vi "rs3 Set Advanced Depth.vi"(0 "Depth Presets":T1(ring), 1 "device in":u64=370866768, 3 "error in (no error)":errorcluster) -> (4 "Set advanced error":string, 5 "Dev out":u64=370866768, 6 "error out":errorcluster)   [LabVIEW 2017, in "libRealSense3.lvlib"]
doc: "The RealSense D4xx cameras are based on a stereo algorithm that has been accelerated as a fixed-function inside an ASIC. There are many parameters that affect the calculation of the depth. The basic task is to solve the correspondance problem - i.e. figure out which patches in the left image match up to those in the right image by doing a search along an epipolar line (x-axis). The x-axis difference for each object point is known as the disparity. \n\nIn general depth can be estimated for most points in the scene, but some points will have a very low confidence because 1. they are may be occluded (not seen by both imagers), or 2. have very little texture on them which will lead to an ambiquity (ex. when looking at a completely uniform white wall it, there are no best correspondances).\n\nThis VI allows you to set the many parameters that affect the algorith, as well as the color reproduction. \nNote that the color correction matrix will NOT have any effect on the depth calculations."
uses:
  libRealSense3.lvlib
panel:
  # "RS3 Set Advanced Depth"
  # "(C) 2020 Intel Corp.,  AGJ"
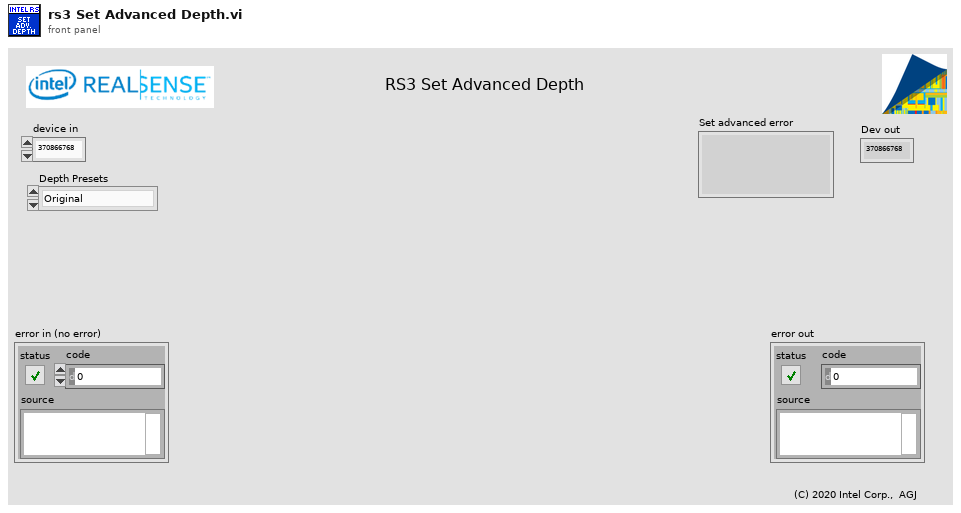
[diagram p1: front panel]
types:
  T1 = enum16{"Original", "High Density", "Medium Density", "High Accuracy", "Hand", "Short Range", "Flat wall"}
  T2 = cluster{"lambdaCensus":sgl, "lambdaAD":sgl, "ignoreSAD":u32}
  T3 = cluster{"depth control":cluster{"plusIncrement":u32, "MinusDecrement":u32, "deepSeaMedianThreshold":u32, "scoreThreshA":u32, "scoreThreshB":u32, "textureDifferenceThreshold":u32, "textureCountThreshold":u32, "deepSeaSecondPeakThreshold":u32, "deepSeaNeighborThreshold":u32, "IrAgreeThreshold":u32}, "STColorCorrection output":cluster{"colorCorrection 1":sgl, "colorCorrection 2":sgl, "colorCorrection 3":sgl, "colorCorrection 4":sgl, "colorCorrection 5":sgl, "colorCorrection 6":sgl, "colorCorrection 7":sgl, "colorCorrection 8":sgl, "colorCorrection 9":sgl, "colorCorrection 10":sgl, "colorCorrection 11":sgl, "colorCorrection 12":sgl}, "HDAD":cluster{"lambdaCensus":sgl, "lambdaAD":sgl, "ignoreSAD":u32}, "ST RSM":cluster{"rsmBypass":u32, "diffThresh":sgl, "sloRauDiffThresh":sgl, "removeThresh":u32}, "ST SLO Penalty":cluster{"sloK1Penalty":u32, "sloK2Penalty":u32, "sloK1PenaltyMod1":u32, "sloK2PenaltyMod1":u32, "sloK1PenaltyMod2":u32, "sloK2PenaltyMod2":u32}, "ST SLO Threshold":cluster{"SLOdiffThresholdRed":u32, "SLODiffThresholdGreen":u32, "SLODiffThresholdBlue":u32}, "ST Rau Threshold":cluster{"rauDiffThresholdRed":u32, "rauDiffThresholdGreen":u32, "rauDiffThresholdBlue":u32}, "ST Color Control":cluster{"disableSADColor":u32, "disableRAUColor":u32, "disableSLORightColor":u32, "disableSLOLeftColor":u32, "disableSADNormalize":u32}, "ST RAU vector":cluster{"minWest":u32, "minEast":u32, "minWEsum":u32, "minNorth":u32, "minSouth":u32, "minNSSum":u32, "uStrink":u32, "vShrink":u32}, "Depth Table":cluster{"depthUnits, um":u32, "depthClampMin":u32, "depthClampMax":u32, "disparityMultiplier":u32, "disparityShift":u32}, "ST_AE_Control":cluster{"meanIntensitySetpoint":u32}, "ST_CensusEnable":cluster{"uDiameter":u32, "vDiameter":u32}}
  T4 = cluster{"depthUnits, um":u32, "depthClampMin":u32, "depthClampMax":u32, "disparityMultiplier":u32, "disparityShift(0-127)":u32}
  T5 = cluster{"minWest (60)":u32, "minEast (61)":u32, "minWEsum (62)":u32, "minNorth (63)":u32, "minSouth (64)":u32, "minNSSum(65)":u32, "uStrink (66)":u32, "vShrink (67)":u32}
  T6 = cluster{"rauDiffThreshRed(73)":u32, "rauDiffThreshGreen(74)":u32, "rauDiffThreshBlue(75)":u32}
  T7 = cluster{"sloK1Penalty (79)":u32, "sloK2Penalty (80)":u32, "sloK1PenaltyMod1(81)":u32, "sloK2PenaltyMod1(82)":u32, "sloK1PenaltyMod2(83)":u32, "sloK2PenaltyMod2(84)":u32}
  T8 = cluster{"SLOdiffThreshRed(76)":u32, "SLODiffThreshGreen(77)":u32, "SLODiffThreshBlue(78)":u32}
  T9 = cluster{"disableSADColor(68)":u32, "disableRAUColor(69)":u32, "disableSLORightColor(70)":u32, "disableSLOLeftColor(71)":u32, "disableSADNormalize(72)":u32}
  T10 = cluster{"rsmBypass (56)":u32, "diffThresh (57)":sgl, "sloRauDiffThresh(58)":sgl, "removeThresh(59)":u32}
  T11 = cluster{"plusIncrement (47)":u32, "MinusDecrement (46)":u32, "deepSeaMedianThreshold (48)":u32, "scoreThreshA(49)":u32, "scoreThreshB (50)":u32, "textureDifferenceThreshold (52)":u32, "textureCountThreshold (51)":u32, "deepSea2ndPeakThresh.(53)":u32, "deepSeaNeighborThresh.(54)":u32, "LRAgreeThreshold (55)":u32}
  T12 = cluster{"plusIncrement":u32, "MinusDecrement":u32, "deepSeaMedianThreshold":u32, "scoreThreshA":u32, "scoreThreshB":u32, "textureDifferenceThreshold":u32, "textureCountThreshold":u32, "deepSeaSecondPeakThreshold":u32, "deepSeaNeighborThreshold":u32, "IrAgreeThreshold":u32}
  T13 = cluster{"rsmBypass":u32, "diffThresh":sgl, "sloRauDiffThresh":sgl, "removeThresh":u32}
  T14 = cluster{"sloK1Penalty":u32, "sloK2Penalty":u32, "sloK1PenaltyMod1":u32, "sloK2PenaltyMod1":u32, "sloK1PenaltyMod2":u32, "sloK2PenaltyMod2":u32}
  T15 = cluster{"SLOdiffThresholdRed":u32, "SLODiffThresholdGreen":u32, "SLODiffThresholdBlue":u32}
  T16 = cluster{"rauDiffThresholdRed":u32, "rauDiffThresholdGreen":u32, "rauDiffThresholdBlue":u32}
  T17 = cluster{"disableSADColor":u32, "disableRAUColor":u32, "disableSLORightColor":u32, "disableSLOLeftColor":u32, "disableSADNormalize":u32}
  T18 = cluster{"minWest":u32, "minEast":u32, "minWEsum":u32, "minNorth":u32, "minSouth":u32, "minNSSum":u32, "uStrink":u32, "vShrink":u32}
  T19 = cluster{"depthUnits, um":u32, "depthClampMin":u32, "depthClampMax":u32, "disparityMultiplier":u32, "disparityShift":u32}
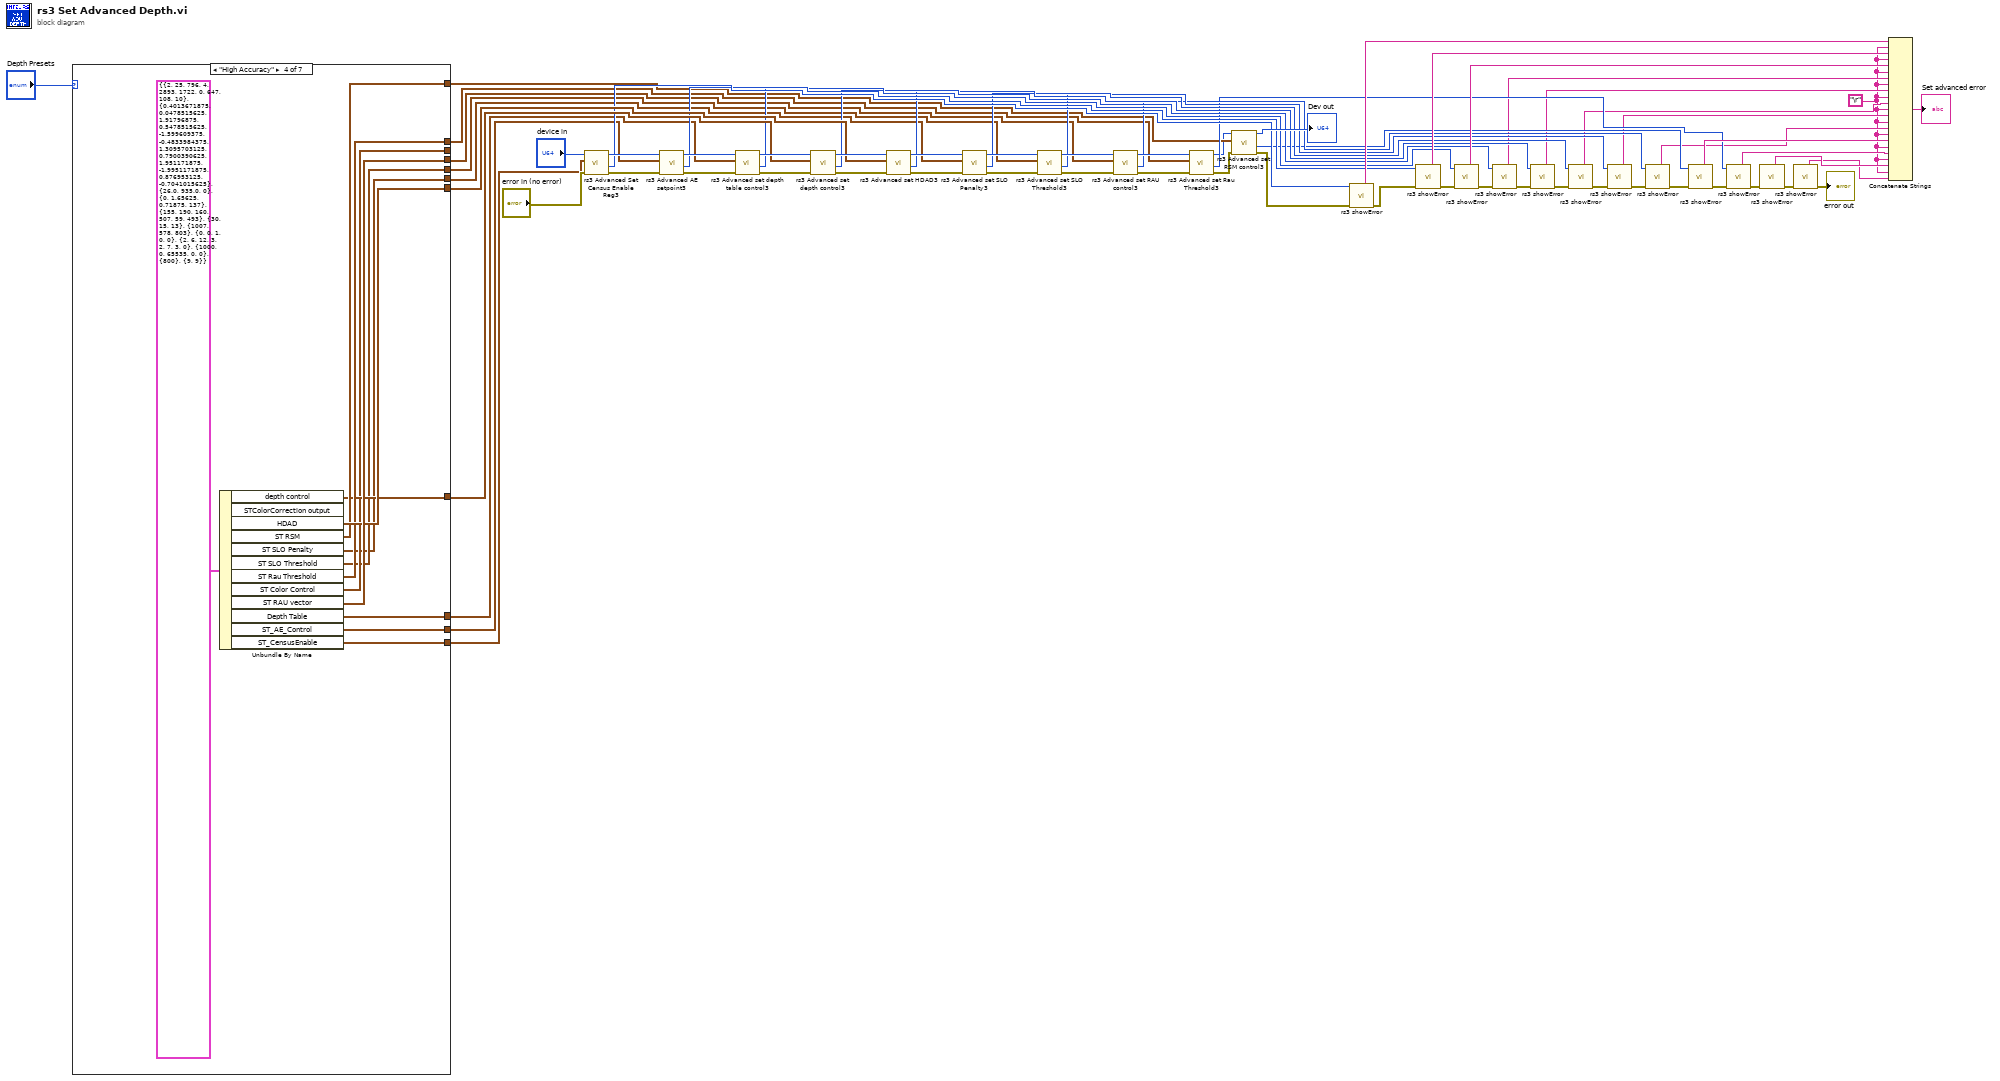
[diagram p0: block diagram]
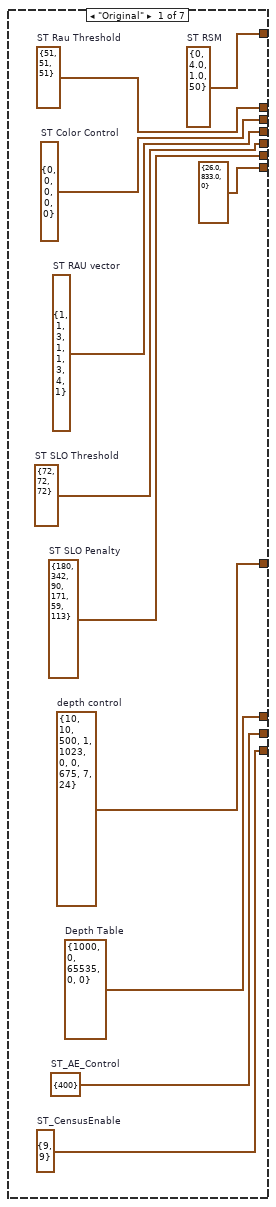
[diagram p2: hidden frame]
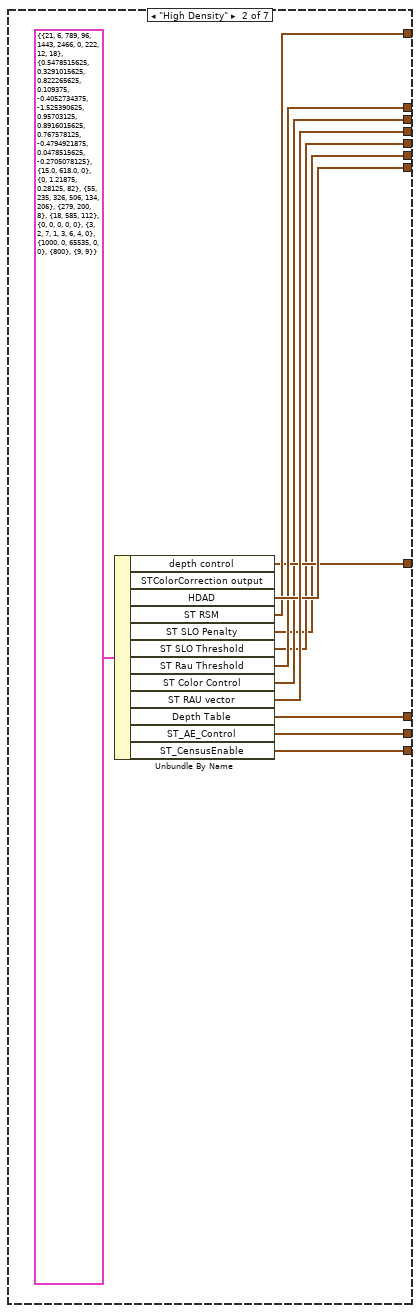
[diagram p3: hidden frame]
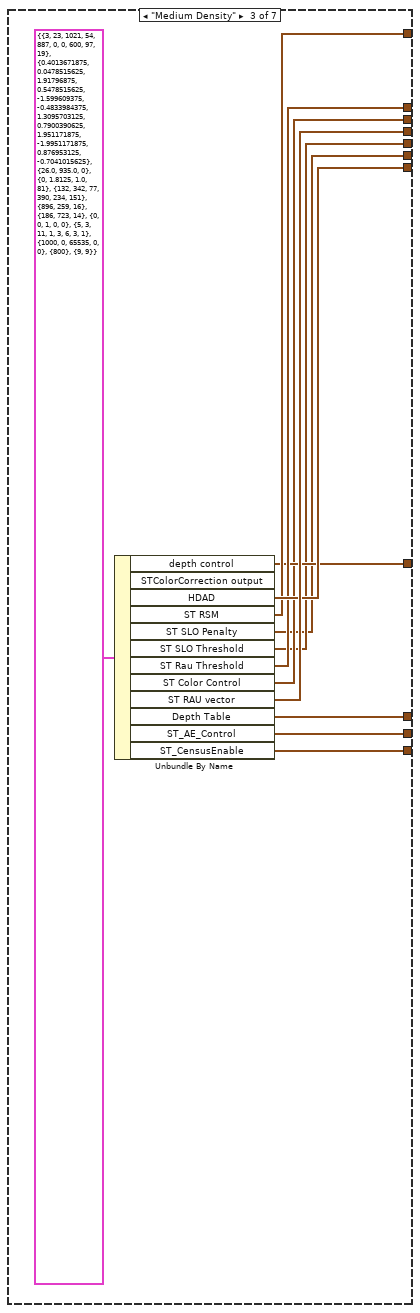
[diagram p4: hidden frame]
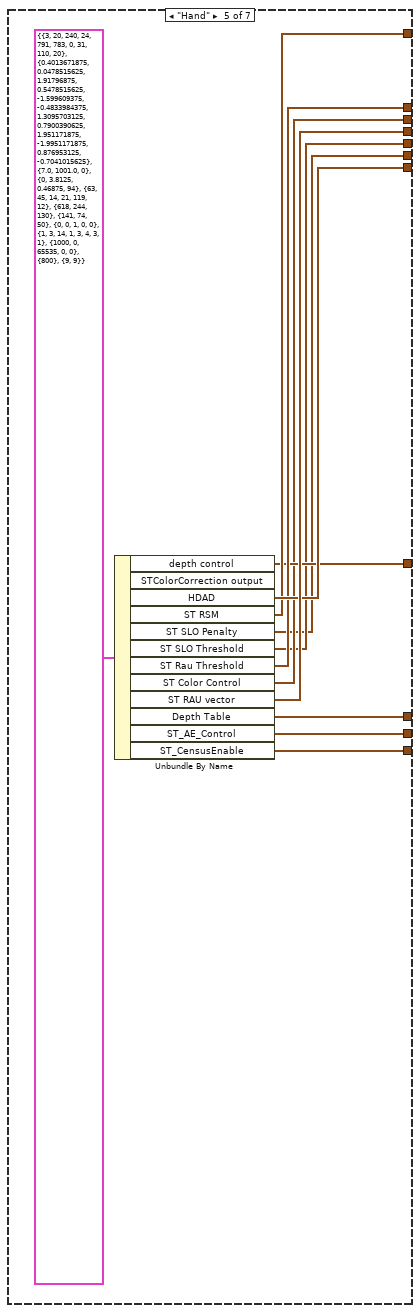
[diagram p5: hidden frame]
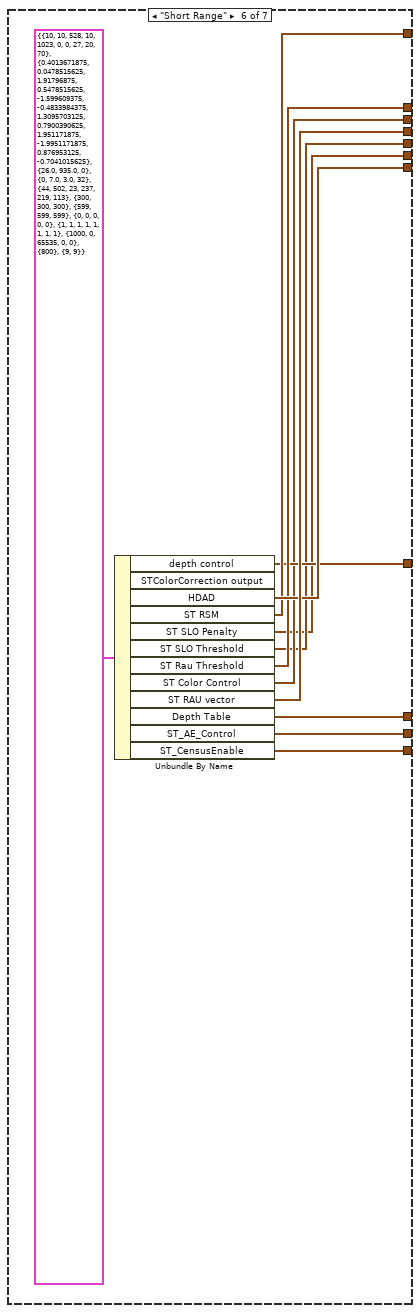
[diagram p6: hidden frame]
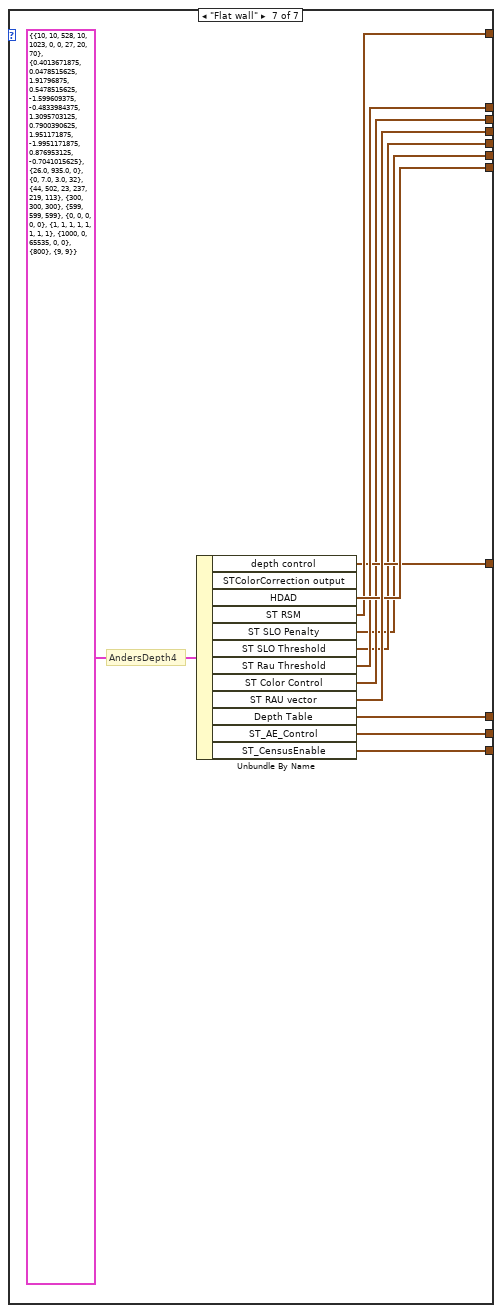
[diagram p7: hidden frame]
diagram:
  w25 = "\r"
  n1 = case shown="\"High Accuracy\"" "Depth Presets" {
    tunnel: [w79 w84 w97 w109 w121 w133 w145] -> w49
    tunnel: [w78 w89 w102 w114 w126 w138 w150] -> w19
    tunnel: [w73 w91 w104 w116 w128 w140 w152] -> w20
    tunnel: [w74 w87 w100 w112 w124 w136 w148] -> w21
    tunnel: [w77 w83 w96 w108 w120 w132 w144] -> _
    tunnel: [w76 w82 w95 w107 w119 w131 w143] -> w22
    tunnel: [w75 w81 w94 w106 w118 w130 w142] -> w23
    tunnel: [T2 {"lambdaCensus"=26.0, "lambdaAD"=833.0, "ignoreSAD"=0} ("HDAD 2") w90 w103 w115 w127 w139 w151] -> w48
    tunnel: [w70 w85 w98 w110 w122 w134 w146] -> w17
    tunnel: [w71 w86 w99 w111 w123 w135 w147] -> w18
    tunnel: [w72 w88 w101 w113 w125 w137 w149] -> w16
    frame "Original" {
      w71 = cluster{"uDiameter":u32, "vDiameter":u32} {"uDiameter"=9, "vDiameter"=9}  # ST_CensusEnable
      w72 = T4 {"depthUnits, um"=1000, "depthClampMin"=0, "depthClampMax"=65535, "disparityMultiplier"=0, "disparityShift(0-127)"=0}  # Depth Table
      w70 = cluster{"meanIntensitySetpoint":u32} {"meanIntensitySetpoint"=400}  # ST_AE_Control
      w73 = T5 {"minWest (60)"=1, "minEast (61)"=1, "minWEsum (62)"=3, "minNorth (63)"=1, "minSouth (64)"=1, "minNSSum(65)"=3, "uStrink (66)"=4, "vShrink (67)"=1}  # ST RAU vector
      w74 = T6 {"rauDiffThreshRed(73)"=51, "rauDiffThreshGreen(74)"=51, "rauDiffThreshBlue(75)"=51}  # ST Rau Threshold
      w75 = T7 {"sloK1Penalty (79)"=180, "sloK2Penalty (80)"=342, "sloK1PenaltyMod1(81)"=90, "sloK2PenaltyMod1(82)"=171, "sloK1PenaltyMod2(83)"=59, "sloK2PenaltyMod2(84)"=113}  # ST SLO Penalty
      w76 = T8 {"SLOdiffThreshRed(76)"=72, "SLODiffThreshGreen(77)"=72, "SLODiffThreshBlue(78)"=72}  # ST SLO Threshold
      w77 = T9 {"disableSADColor(68)"=0, "disableRAUColor(69)"=0, "disableSLORightColor(70)"=0, "disableSLOLeftColor(71)"=0, "disableSADNormalize(72)"=0}  # ST Color Control
      w78 = T10 {"rsmBypass (56)"=0, "diffThresh (57)"=4.0, "sloRauDiffThresh(58)"=1.0, "removeThresh(59)"=50}  # ST RSM
      w79 = T11 {"plusIncrement (47)"=10, "MinusDecrement (46)"=10, "deepSeaMedianThreshold (48)"=500, "scoreThreshA(49)"=1, "scoreThreshB (50)"=1023, "textureDifferenceThreshold (52)"=0, "textureCountThreshold (51)"=0, "deepSea2ndPeakThresh.(53)"=675, "deepSeaNeighborThresh.(54)"=7, "LRAgreeThreshold (55)"=24}  # depth control
    }
    frame "High Density" {
      n2 = Unbundle By Name(T3 {"depth control"={"plusIncrement"=21, "MinusDecrement"=6, "deepSeaMedianThreshold"=789, "scoreThreshA"=96, "scoreThreshB"=1443, "textureDifferenceThreshold"=2466, "textureCountThreshold"=0, "deepSeaSecondPeakThreshold"=222, "deepSeaNeighborThreshold"=12, "IrAgreeThreshold"=18}, "STColorCorrection output"={"colorCorrection 1"=0.54785156, "colorCorrection 2"=0.32910156, "colorCorrection 3"=0.8222656, "colorCorrection 4"=0.109375, "colorCorrection 5"=-0.40527344, "colorCorrection 6"=-1.5253906, "colorCorrection 7"=0.95703125, "colorCorrection 8"=0.89160156, "colorCorrection 9"=0.7675781, "colorCorrection 10"=-0.4794922, "colorCorrection 11"=0.047851562, "colorCorrection 12"=-0.2705078}, "HDAD"={"lambdaCensus"=15.0, "lambdaAD"=618.0, "ignoreSAD"=0}, "ST RSM"={"rsmBypass"=0, "diffThresh"=1.21875, "sloRauDiffThresh"=0.28125, "removeThresh"=82}, "ST SLO Penalty"={"sloK1Penalty"=55, "sloK2Penalty"=235, "sloK1PenaltyMod1"=326, "sloK2PenaltyMod1"=506, "sloK1PenaltyMod2"=134, "sloK2PenaltyMod2"=206}, "ST SLO Threshold"={"SLOdiffThresholdRed"=279, "SLODiffThresholdGreen"=200, "SLODiffThresholdBlue"=8}, "ST Rau Threshold"={"rauDiffThresholdRed"=18, "rauDiffThresholdGreen"=585, "rauDiffThresholdBlue"=112}, "ST Color Control"={"disableSADColor"=0, "disableRAUColor"=0, "disableSLORightColor"=0, "disableSLOLeftColor"=0, "disableSADNormalize"=0}, "ST RAU vector"={"minWest"=3, "minEast"=2, "minWEsum"=7, "minNorth"=1, "minSouth"=3, "minNSSum"=6, "uStrink"=4, "vShrink"=0}, "Depth Table"={"depthUnits, um"=1000, "depthClampMin"=0, "depthClampMax"=65535, "disparityMultiplier"=0, "disparityShift"=0}, "ST_AE_Control"={"meanIntensitySetpoint"=800}, "ST_CensusEnable"={"uDiameter"=9, "vDiameter"=9}} ("depth settings 2")) -> ("depth control"=w84:T12, "HDAD"=w90:T2, "ST RSM"=w89:T13, "ST SLO Penalty"=w81:T14, "ST SLO Threshold"=w82:T15, "ST Rau Threshold"=w87:T16, "ST Color Control"=w83:T17, "ST RAU vector"=w91:T18, "Depth Table"=w88:T19, "ST_AE_Control"=w85:cluster{"meanIntensitySetpoint":u32}, "ST_CensusEnable"=w86:cluster{"uDiameter":u32, "vDiameter":u32})  [unwired: 1 out]
    }
    frame "Medium Density" {
      n3 = Unbundle By Name(T3 {"depth control"={"plusIncrement"=3, "MinusDecrement"=23, "deepSeaMedianThreshold"=1021, "scoreThreshA"=54, "scoreThreshB"=887, "textureDifferenceThreshold"=0, "textureCountThreshold"=0, "deepSeaSecondPeakThreshold"=600, "deepSeaNeighborThreshold"=97, "IrAgreeThreshold"=19}, "STColorCorrection output"={"colorCorrection 1"=0.4013672, "colorCorrection 2"=0.047851562, "colorCorrection 3"=1.9179688, "colorCorrection 4"=0.54785156, "colorCorrection 5"=-1.5996094, "colorCorrection 6"=-0.48339844, "colorCorrection 7"=1.3095703, "colorCorrection 8"=0.79003906, "colorCorrection 9"=1.9511719, "colorCorrection 10"=-1.9951172, "colorCorrection 11"=0.8769531, "colorCorrection 12"=-0.70410156}, "HDAD"={"lambdaCensus"=26.0, "lambdaAD"=935.0, "ignoreSAD"=0}, "ST RSM"={"rsmBypass"=0, "diffThresh"=1.8125, "sloRauDiffThresh"=1.0, "removeThresh"=81}, "ST SLO Penalty"={"sloK1Penalty"=132, "sloK2Penalty"=342, "sloK1PenaltyMod1"=77, "sloK2PenaltyMod1"=390, "sloK1PenaltyMod2"=234, "sloK2PenaltyMod2"=151}, "ST SLO Threshold"={"SLOdiffThresholdRed"=896, "SLODiffThresholdGreen"=259, "SLODiffThresholdBlue"=16}, "ST Rau Threshold"={"rauDiffThresholdRed"=186, "rauDiffThresholdGreen"=723, "rauDiffThresholdBlue"=14}, "ST Color Control"={"disableSADColor"=0, "disableRAUColor"=0, "disableSLORightColor"=1, "disableSLOLeftColor"=0, "disableSADNormalize"=0}, "ST RAU vector"={"minWest"=5, "minEast"=3, "minWEsum"=11, "minNorth"=1, "minSouth"=3, "minNSSum"=6, "uStrink"=3, "vShrink"=1}, "Depth Table"={"depthUnits, um"=1000, "depthClampMin"=0, "depthClampMax"=65535, "disparityMultiplier"=0, "disparityShift"=0}, "ST_AE_Control"={"meanIntensitySetpoint"=800}, "ST_CensusEnable"={"uDiameter"=9, "vDiameter"=9}} ("depth settings 2")) -> ("depth control"=w97:T12, "HDAD"=w103:T2, "ST RSM"=w102:T13, "ST SLO Penalty"=w94:T14, "ST SLO Threshold"=w95:T15, "ST Rau Threshold"=w100:T16, "ST Color Control"=w96:T17, "ST RAU vector"=w104:T18, "Depth Table"=w101:T19, "ST_AE_Control"=w98:cluster{"meanIntensitySetpoint":u32}, "ST_CensusEnable"=w99:cluster{"uDiameter":u32, "vDiameter":u32})  [unwired: 1 out]
    }
    frame "High Accuracy" {
      n4 = Unbundle By Name(T3 {"depth control"={"plusIncrement"=2, "MinusDecrement"=25, "deepSeaMedianThreshold"=796, "scoreThreshA"=4, "scoreThreshB"=2893, "textureDifferenceThreshold"=1722, "textureCountThreshold"=0, "deepSeaSecondPeakThreshold"=647, "deepSeaNeighborThreshold"=108, "IrAgreeThreshold"=10}, "STColorCorrection output"={"colorCorrection 1"=0.4013672, "colorCorrection 2"=0.047851562, "colorCorrection 3"=1.9179688, "colorCorrection 4"=0.54785156, "colorCorrection 5"=-1.5996094, "colorCorrection 6"=-0.48339844, "colorCorrection 7"=1.3095703, "colorCorrection 8"=0.79003906, "colorCorrection 9"=1.9511719, "colorCorrection 10"=-1.9951172, "colorCorrection 11"=0.8769531, "colorCorrection 12"=-0.70410156}, "HDAD"={"lambdaCensus"=26.0, "lambdaAD"=935.0, "ignoreSAD"=0}, "ST RSM"={"rsmBypass"=0, "diffThresh"=1.65625, "sloRauDiffThresh"=0.71875, "removeThresh"=137}, "ST SLO Penalty"={"sloK1Penalty"=155, "sloK2Penalty"=190, "sloK1PenaltyMod1"=160, "sloK2PenaltyMod1"=507, "sloK1PenaltyMod2"=59, "sloK2PenaltyMod2"=493}, "ST SLO Threshold"={"SLOdiffThresholdRed"=30, "SLODiffThresholdGreen"=15, "SLODiffThresholdBlue"=13}, "ST Rau Threshold"={"rauDiffThresholdRed"=1007, "rauDiffThresholdGreen"=578, "rauDiffThresholdBlue"=803}, "ST Color Control"={"disableSADColor"=0, "disableRAUColor"=0, "disableSLORightColor"=1, "disableSLOLeftColor"=0, "disableSADNormalize"=0}, "ST RAU vector"={"minWest"=2, "minEast"=6, "minWEsum"=12, "minNorth"=3, "minSouth"=2, "minNSSum"=7, "uStrink"=3, "vShrink"=0}, "Depth Table"={"depthUnits, um"=1000, "depthClampMin"=0, "depthClampMax"=65535, "disparityMultiplier"=0, "disparityShift"=0}, "ST_AE_Control"={"meanIntensitySetpoint"=800}, "ST_CensusEnable"={"uDiameter"=9, "vDiameter"=9}} ("depth settings 2")) -> ("depth control"=w109:T12, "HDAD"=w115:T2, "ST RSM"=w114:T13, "ST SLO Penalty"=w106:T14, "ST SLO Threshold"=w107:T15, "ST Rau Threshold"=w112:T16, "ST Color Control"=w108:T17, "ST RAU vector"=w116:T18, "Depth Table"=w113:T19, "ST_AE_Control"=w110:cluster{"meanIntensitySetpoint":u32}, "ST_CensusEnable"=w111:cluster{"uDiameter":u32, "vDiameter":u32})  [unwired: 1 out]
    }
    frame "Hand" {
      n5 = Unbundle By Name(T3 {"depth control"={"plusIncrement"=3, "MinusDecrement"=20, "deepSeaMedianThreshold"=240, "scoreThreshA"=24, "scoreThreshB"=791, "textureDifferenceThreshold"=783, "textureCountThreshold"=0, "deepSeaSecondPeakThreshold"=31, "deepSeaNeighborThreshold"=110, "IrAgreeThreshold"=20}, "STColorCorrection output"={"colorCorrection 1"=0.4013672, "colorCorrection 2"=0.047851562, "colorCorrection 3"=1.9179688, "colorCorrection 4"=0.54785156, "colorCorrection 5"=-1.5996094, "colorCorrection 6"=-0.48339844, "colorCorrection 7"=1.3095703, "colorCorrection 8"=0.79003906, "colorCorrection 9"=1.9511719, "colorCorrection 10"=-1.9951172, "colorCorrection 11"=0.8769531, "colorCorrection 12"=-0.70410156}, "HDAD"={"lambdaCensus"=7.0, "lambdaAD"=1001.0, "ignoreSAD"=0}, "ST RSM"={"rsmBypass"=0, "diffThresh"=3.8125, "sloRauDiffThresh"=0.46875, "removeThresh"=94}, "ST SLO Penalty"={"sloK1Penalty"=63, "sloK2Penalty"=45, "sloK1PenaltyMod1"=14, "sloK2PenaltyMod1"=21, "sloK1PenaltyMod2"=119, "sloK2PenaltyMod2"=12}, "ST SLO Threshold"={"SLOdiffThresholdRed"=618, "SLODiffThresholdGreen"=244, "SLODiffThresholdBlue"=130}, "ST Rau Threshold"={"rauDiffThresholdRed"=141, "rauDiffThresholdGreen"=74, "rauDiffThresholdBlue"=50}, "ST Color Control"={"disableSADColor"=0, "disableRAUColor"=0, "disableSLORightColor"=1, "disableSLOLeftColor"=0, "disableSADNormalize"=0}, "ST RAU vector"={"minWest"=1, "minEast"=3, "minWEsum"=14, "minNorth"=1, "minSouth"=3, "minNSSum"=4, "uStrink"=3, "vShrink"=1}, "Depth Table"={"depthUnits, um"=1000, "depthClampMin"=0, "depthClampMax"=65535, "disparityMultiplier"=0, "disparityShift"=0}, "ST_AE_Control"={"meanIntensitySetpoint"=800}, "ST_CensusEnable"={"uDiameter"=9, "vDiameter"=9}} ("depth settings 2")) -> ("depth control"=w121:T12, "HDAD"=w127:T2, "ST RSM"=w126:T13, "ST SLO Penalty"=w118:T14, "ST SLO Threshold"=w119:T15, "ST Rau Threshold"=w124:T16, "ST Color Control"=w120:T17, "ST RAU vector"=w128:T18, "Depth Table"=w125:T19, "ST_AE_Control"=w122:cluster{"meanIntensitySetpoint":u32}, "ST_CensusEnable"=w123:cluster{"uDiameter":u32, "vDiameter":u32})  [unwired: 1 out]
    }
    frame "Short Range" {
      n6 = Unbundle By Name(T3 {"depth control"={"plusIncrement"=10, "MinusDecrement"=10, "deepSeaMedianThreshold"=528, "scoreThreshA"=10, "scoreThreshB"=1023, "textureDifferenceThreshold"=0, "textureCountThreshold"=0, "deepSeaSecondPeakThreshold"=27, "deepSeaNeighborThreshold"=20, "IrAgreeThreshold"=70}, "STColorCorrection output"={"colorCorrection 1"=0.4013672, "colorCorrection 2"=0.047851562, "colorCorrection 3"=1.9179688, "colorCorrection 4"=0.54785156, "colorCorrection 5"=-1.5996094, "colorCorrection 6"=-0.48339844, "colorCorrection 7"=1.3095703, "colorCorrection 8"=0.79003906, "colorCorrection 9"=1.9511719, "colorCorrection 10"=-1.9951172, "colorCorrection 11"=0.8769531, "colorCorrection 12"=-0.70410156}, "HDAD"={"lambdaCensus"=26.0, "lambdaAD"=935.0, "ignoreSAD"=0}, "ST RSM"={"rsmBypass"=0, "diffThresh"=7.0, "sloRauDiffThresh"=3.0, "removeThresh"=32}, "ST SLO Penalty"={"sloK1Penalty"=44, "sloK2Penalty"=502, "sloK1PenaltyMod1"=23, "sloK2PenaltyMod1"=237, "sloK1PenaltyMod2"=219, "sloK2PenaltyMod2"=113}, "ST SLO Threshold"={"SLOdiffThresholdRed"=300, "SLODiffThresholdGreen"=300, "SLODiffThresholdBlue"=300}, "ST Rau Threshold"={"rauDiffThresholdRed"=599, "rauDiffThresholdGreen"=599, "rauDiffThresholdBlue"=599}, "ST Color Control"={"disableSADColor"=0, "disableRAUColor"=0, "disableSLORightColor"=0, "disableSLOLeftColor"=0, "disableSADNormalize"=0}, "ST RAU vector"={"minWest"=1, "minEast"=1, "minWEsum"=1, "minNorth"=1, "minSouth"=1, "minNSSum"=1, "uStrink"=1, "vShrink"=1}, "Depth Table"={"depthUnits, um"=1000, "depthClampMin"=0, "depthClampMax"=65535, "disparityMultiplier"=0, "disparityShift"=0}, "ST_AE_Control"={"meanIntensitySetpoint"=800}, "ST_CensusEnable"={"uDiameter"=9, "vDiameter"=9}} ("depth settings 2")) -> ("depth control"=w133:T12, "HDAD"=w139:T2, "ST RSM"=w138:T13, "ST SLO Penalty"=w130:T14, "ST SLO Threshold"=w131:T15, "ST Rau Threshold"=w136:T16, "ST Color Control"=w132:T17, "ST RAU vector"=w140:T18, "Depth Table"=w137:T19, "ST_AE_Control"=w134:cluster{"meanIntensitySetpoint":u32}, "ST_CensusEnable"=w135:cluster{"uDiameter":u32, "vDiameter":u32})  [unwired: 1 out]
    }
    frame "Flat wall" {
      # "AndersDepth4"
      n7 = Unbundle By Name(T3 {"depth control"={"plusIncrement"=10, "MinusDecrement"=10, "deepSeaMedianThreshold"=528, "scoreThreshA"=10, "scoreThreshB"=1023, "textureDifferenceThreshold"=0, "textureCountThreshold"=0, "deepSeaSecondPeakThreshold"=27, "deepSeaNeighborThreshold"=20, "IrAgreeThreshold"=70}, "STColorCorrection output"={"colorCorrection 1"=0.4013672, "colorCorrection 2"=0.047851562, "colorCorrection 3"=1.9179688, "colorCorrection 4"=0.54785156, "colorCorrection 5"=-1.5996094, "colorCorrection 6"=-0.48339844, "colorCorrection 7"=1.3095703, "colorCorrection 8"=0.79003906, "colorCorrection 9"=1.9511719, "colorCorrection 10"=-1.9951172, "colorCorrection 11"=0.8769531, "colorCorrection 12"=-0.70410156}, "HDAD"={"lambdaCensus"=26.0, "lambdaAD"=935.0, "ignoreSAD"=0}, "ST RSM"={"rsmBypass"=0, "diffThresh"=7.0, "sloRauDiffThresh"=3.0, "removeThresh"=32}, "ST SLO Penalty"={"sloK1Penalty"=44, "sloK2Penalty"=502, "sloK1PenaltyMod1"=23, "sloK2PenaltyMod1"=237, "sloK1PenaltyMod2"=219, "sloK2PenaltyMod2"=113}, "ST SLO Threshold"={"SLOdiffThresholdRed"=300, "SLODiffThresholdGreen"=300, "SLODiffThresholdBlue"=300}, "ST Rau Threshold"={"rauDiffThresholdRed"=599, "rauDiffThresholdGreen"=599, "rauDiffThresholdBlue"=599}, "ST Color Control"={"disableSADColor"=0, "disableRAUColor"=0, "disableSLORightColor"=0, "disableSLOLeftColor"=0, "disableSADNormalize"=0}, "ST RAU vector"={"minWest"=1, "minEast"=1, "minWEsum"=1, "minNorth"=1, "minSouth"=1, "minNSSum"=1, "uStrink"=1, "vShrink"=1}, "Depth Table"={"depthUnits, um"=1000, "depthClampMin"=0, "depthClampMax"=65535, "disparityMultiplier"=0, "disparityShift"=0}, "ST_AE_Control"={"meanIntensitySetpoint"=800}, "ST_CensusEnable"={"uDiameter"=9, "vDiameter"=9}} ("depth settings 2")) -> ("depth control"=w145:T12, "HDAD"=w151:T2, "ST RSM"=w150:T13, "ST SLO Penalty"=w142:T14, "ST SLO Threshold"=w143:T15, "ST Rau Threshold"=w148:T16, "ST Color Control"=w144:T17, "ST RAU vector"=w152:T18, "Depth Table"=w149:T19, "ST_AE_Control"=w146:cluster{"meanIntensitySetpoint":u32}, "ST_CensusEnable"=w147:cluster{"uDiameter":u32, "vDiameter":u32})  [unwired: 1 out]
    }
  }
  n8 = call "rs3 Advanced Set Census Enable Reg3.vi"("error in (no error)"="error in (no error)", "ST_CensusEnableReg"=w18, "device in"="device in") -> ("error out 2"=w67:errorcluster, "error"=w45:u64, "Dev out"=w66:u64)  [unwired: 6 in]
  n9 = call "rs3 Advanced AE setpoint3.vi"("error in (no error)"=w67, "ST_AE_Control"=w17, "device in"=w66) -> ("error out"=w65:errorcluster, "error"=w43:u64, "Dev out"=w64:u64)  [unwired: 6 in]
  n10 = call "rs3 Advanced set depth table control3.vi"("error in (no error)"=w65, "Depth Table"=w16, "device in"=w64) -> ("error out 2"=w63:errorcluster, "error"=w41:u64, "Dev out"=w62:u64)  [unwired: 6 in]
  n11 = call "rs3 Advanced set depth control3.vi"("error in (no error)"=w63, "depth control"=w49, "device in"=w62) -> ("error out"=w61:errorcluster, "error"=w39:u64, "Dev out"=w60:u64)  [unwired: 6 in]
  n12 = call "rs3 Advanced set HDAD3.vi"("error in (no error)"=w61, "HDAD"=w48, "device in"=w60) -> ("error out"=w59:errorcluster, "error"=w38:u64, "Dev out"=w58:u64)  [unwired: 6 in]
  n13 = call "rs3 Advanced set SLO Penalty3.vi"("error in (no error)"=w59, "ST SLO Penalty"=w23, "device in"=w58) -> ("error out"=w57:errorcluster, "error"=w37:u64, "Dev out"=w56:u64)  [unwired: 6 in]
  n14 = call "rs3 Advanced set SLO Threshold3.vi"("error in (no error)"=w57, "ST SLO Threshold"=w22, "device in"=w56) -> ("error out"=w55:errorcluster, "error"=w36:u64, "Dev out"=w54:u64)  [unwired: 6 in]
  n15 = call "rs3 Advanced set RAU control3.vi"("error in (no error)"=w55, "ST RAU vector"=w20, "device in"=w54) -> ("error out"=w53:errorcluster, "error"=w35:u64, "Dev out"=w52:u64)  [unwired: 6 in]
  n16 = call "rs3 Advanced set Rau Threshold3.vi"("error in (no error)"=w53, "ST Rau Threshold"=w21, "device in"=w52) -> ("error out"=w1:errorcluster, "error"=w34:u64, "Dev out"=w2:u64)  [unwired: 6 in]
  n17 = call "rs3 Advanced set RSM control3.vi"("error in (no error)"=w1, "ST RSM"=w19, "device in"=w2) -> ("error out"=w3:errorcluster, "error"=w33:u64, "Dev out"=→"Dev out":u64)  [unwired: 6 in]
  n18 = call "rs3 showError.vi"("error in (no error)"=w3, "error"=w45) -> ("error out"=w15:errorcluster, "Error summary"=w44:string)  [unwired: 5 in, 3 out]
  n19 = call "rs3 showError.vi"("error in (no error)"=w15, "error"=w43) -> ("error out"=w14:errorcluster, "Error summary"=w42:string)  [unwired: 5 in, 3 out]
  n20 = call "rs3 showError.vi"("error in (no error)"=w14, "error"=w41) -> ("error out"=w13:errorcluster, "Error summary"=w40:string)  [unwired: 5 in, 3 out]
  n21 = call "rs3 showError.vi"("error in (no error)"=w13, "error"=w39) -> ("error out"=w12:errorcluster, "Error summary"=w32:string)  [unwired: 5 in, 3 out]
  n22 = call "rs3 showError.vi"("error in (no error)"=w12, "error"=w38) -> ("error out"=w11:errorcluster, "Error summary"=w31:string)  [unwired: 5 in, 3 out]
  n23 = call "rs3 showError.vi"("error in (no error)"=w11, "error"=w37) -> ("error out"=w10:errorcluster, "Error summary"=w30:string)  [unwired: 5 in, 3 out]
  n24 = call "rs3 showError.vi"("error in (no error)"=w10, "error"=w36) -> ("error out"=w9:errorcluster, "Error summary"=w29:string)  [unwired: 5 in, 3 out]
  n25 = call "rs3 showError.vi"("error in (no error)"=w9, "error"=w35) -> ("error out"=w8:errorcluster, "Error summary"=w28:string)  [unwired: 5 in, 3 out]
  n26 = call "rs3 showError.vi"("error in (no error)"=w8, "error"=w33) -> ("error out"=w7:errorcluster, "Error summary"=w47:string)  [unwired: 5 in, 3 out]
  n27 = call "rs3 showError.vi"("error in (no error)"=w7, "error"=w34) -> ("error out"=w6:errorcluster, "Error summary"=w27:string)  [unwired: 5 in, 3 out]
  n28 = call "rs3 showError.vi"("error in (no error)"=w6) -> ("error out"=w5:errorcluster, "Error summary"=w26:string)  [unwired: 6 in, 3 out]
  n29 = call "rs3 showError.vi"("error in (no error)"=w5) -> ("error out"=→"error out":errorcluster, "Error summary"=w24:string)  [unwired: 6 in, 3 out]
  n30 = Concatenate Strings(w44, w25, w42, w25, w40, w25, w32, w25, w31, w25, w30, w25, w29, w25, w28, w25, w47, w25, w27, w25, w26, w25, w24) -> (→"Set advanced error":string)
